vi "DrawWaypoints.vi"(2 "Array":i32[][](array[numeric]), 3 "2D Picture":picture) -> (0 "new picture":picture)   [LabVIEW 2012]
doc: "Draws a magenta circle at the curretn (x,y) coordinates of the Robot in the current mission definition file.\nInputs:\nPicture to draw on\nCluster X\n y coordinates of robot\nOutput:\nmodified picture"
panel:
  in  "color(black)":u32(colorbox)=16318208
  # "Draws a circle at the current x,y coordinates of the robot"
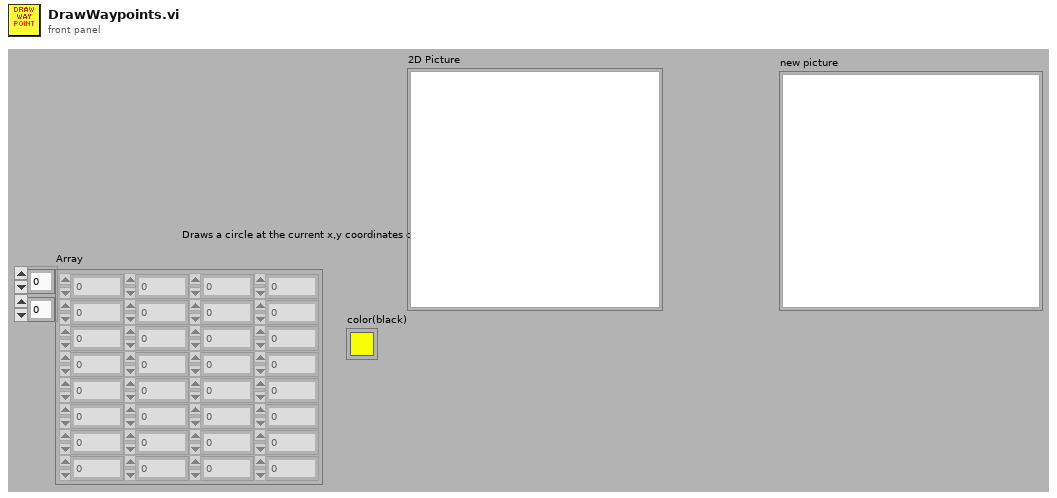
[diagram p1: front panel]
types:
  T1 = cluster{"Width":u16, "Style":enum32{"Solid", "Dash", "Dot", "DashDot", "DashDotDot"}}
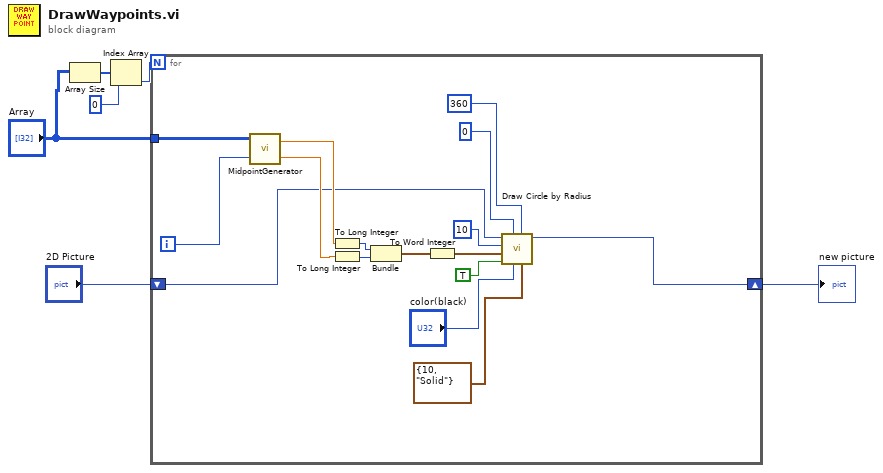
[diagram p0: block diagram]
diagram:
  n1 = Array Size(array="Array") -> (size(s)=w5:i32[])
  n2 = Index Array(array=w5, index=0) -> (element=w3:i32)
  n3 = for {
    N: w3 -> [_]
    tunnel: "Array" -> [w22]
    shift-right: [w7] -> w1
    shift-left: "2D Picture" -> [w8]
    i -> [w21]
    n4 = call "MidpointGenerator.vi"("Waypoint"=w21, "Array"=w22) -> ("Y"=w9:dbl, "X"=w10:dbl)
    n5 = To Long Integer(number=w10) -> (32bit integer=w14:i32)
    n6 = To Long Integer(number=w9) -> (32bit integer=w13:i32)
    n7 = Bundle(w14, w13) -> (w12:cluster{i32, i32})  [unwired: 1 in]
    n8 = To Word Integer(number=w12) -> (16bit integer=w11:cluster{i16, i16})
    n9 = call <vilib>:"Draw Circle by Radius.vi"("pen"=T1 {"Width"=10, "Style"=enum."Solid"}, "arc size(360)"=i16 360, "color(black)"="color(black)", "start angle(0)"=i16 0, "fill?(F)"=TRUE, "pixel center"=w11, "radius"=i16 10, "picture"=w8) -> ("new picture"=w7:picture)  [unwired: 3 in]
  }
  "new picture" <- w1
